vi "MDML_funcx.vi"(6 "connMeta 7":T1, 7 "Experiment ID 3":string, 8 "error in (no error)":errorcluster, 9 "queries":T3[](array[typedef]), 10 "String 2":string, 11 "String":string) -> (0 "error out":errorcluster)   [LabVIEW 2018]
uses:
  query_part.ctl
  Downloads/mqtt_lv2013_201708181938/mqtt_lv2013/mqtt Folder/src/class/mqtt/mqttTypedef/mqttConnectionMeta.ctl
  Downloads/mqtt_lv2013_201708181938/mqtt_lv2013/mqtt Folder/src/class/mqtt/mqttTypedef/mqttQOSlevel.ctl
  funcx_message.ctl
  Downloads/mqtt_lv2013_201708181938/mqtt_lv2013/mqtt Folder/src/class/mqtt/mqtt.lvclass
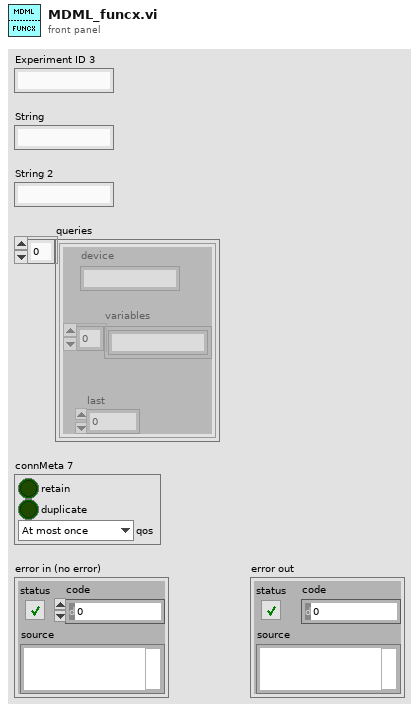
[diagram p1: front panel]
types:
  T1 = typedef "mqttConnectionMeta.ctl" = cluster{"retain":bool, "duplicate":bool, "qos":T2}
  T2 = typedef "mqttQOSlevel.ctl" = enum8{"At most once", "At least once", "Exactly once", "Reserved"}
  T3 = typedef "query_part.ctl" = cluster{"device":string, "last":dbl, "variables":string[]}
  T4 = typedef "funcx_message.ctl" = cluster{"function_id":string, "endpoint_id":string, "timestamp":string, "queries":cluster{"device":string, "last":dbl, "variables":string[]}[]}
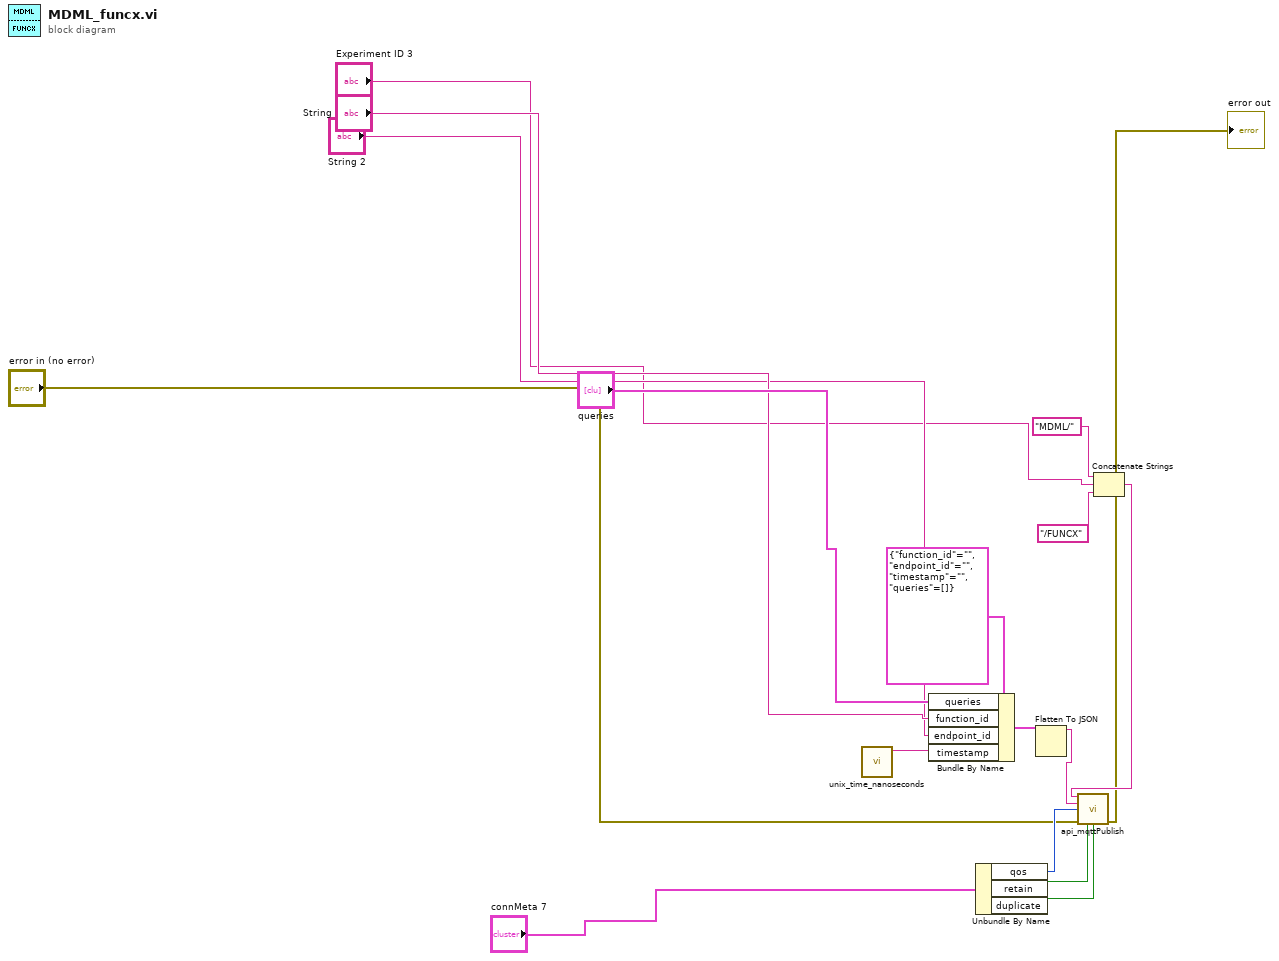
[diagram p0: block diagram]
diagram:
  n1 = call "unix_time_nanoseconds.vi"() -> ("String"=w1:string)  [unwired: 11 in]
  n2 = Bundle By Name(cluster=T4 {"function_id"="", "endpoint_id"="", "timestamp"="", "queries"=[]} ("input cluster"), "queries"="queries", "function_id"="String", "endpoint_id"="String 2", "timestamp"=w1) -> (w16:T4)
  n3 = Unbundle By Name("connMeta 7") -> ("qos"=w11:T2, "retain"=w9:bool, "duplicate"=w10:bool)
  n4 = Flatten To JSON(anything=w16) -> (JSON string=w17:string)  [unwired: 2 in, 1 out]
  n5 = Concatenate Strings("MDML/", "Experiment ID 3", "/FUNCX") -> (w14:string)
  n6 = call "api_mqttPublish.vi"("topic"=w14, "value"=w17, "QoS (At most once)"=w11, "error in (no error)"="error in (no error)", "retain(F)"=w9, "duplicate(F)"=w10) -> ("error out"=→"error out":errorcluster)  [unwired: 8 in, 1 out]
